vi "Format Debug String.vi"(7 "Version":string, 8 "error in (no error)":errorcluster, 9 "State":string, 10 "severity (Informational)":i32(ring)=2 items=["Error", "Warning", "Informational"], 11 "Name":string) -> (0 "error out":errorcluster)   [LabVIEW 2019, in "Instrument Addon Engine.lvlib"]
uses:
  Instrument Addon Engine.lvlib
  <vilib>/Utility/SystemLogging/NI_SystemLogging.lvlib
panel:
  out "Debug String":string
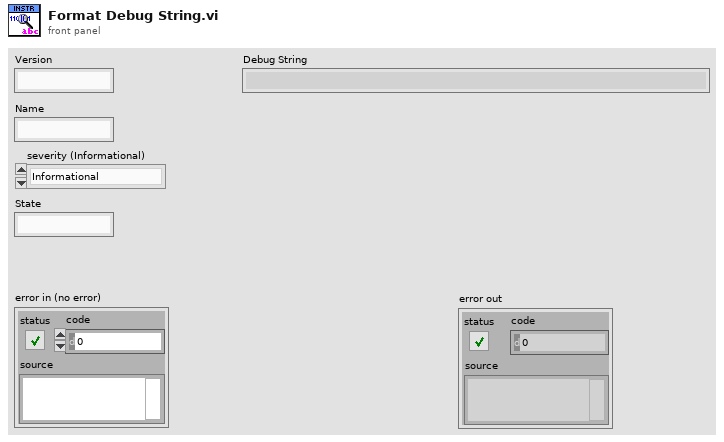
[diagram p1: front panel]
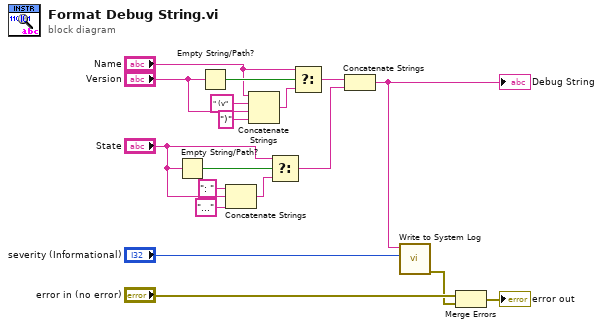
[diagram p0: block diagram]
diagram:
  n1 = Empty String/Path?(string/path="State") -> (empty?=w14:bool)
  n2 = Empty String/Path?(string/path="Version") -> (empty?=w18:bool)
  n3 = Concatenate Strings(": " ("string"), "State", "..." ("string")) -> (w12:string)
  n4 = Concatenate Strings("Name", " (v" ("string"), "Version", ")" ("string")) -> (w15:string)
  n5 = Select(t="State", s=w14, f=w12) -> (s? t:f=w10:string)
  n6 = Select(t="Name", s=w18, f=w15) -> (s? t:f=w7:string)
  n7 = Concatenate Strings(w7, w10) -> (w4:string)
  "Debug String" <- w4
  n8 = call <vilib>:"Write to System Log.vi"("severity"="severity (Informational)", "message"=w4) -> ("error out"=w2:errorcluster)  [unwired: 9 in]
  n9 = Merge Errors("error in (no error)", w2) -> (→"error out":errorcluster)
